vi "FTW-Test-Socket-Stress-InboxShutdown.vi"() -> (0 "Test Result":errorcluster)   [LabVIEW 2015]
panel:
  out "Endpoints":string[](array[string])
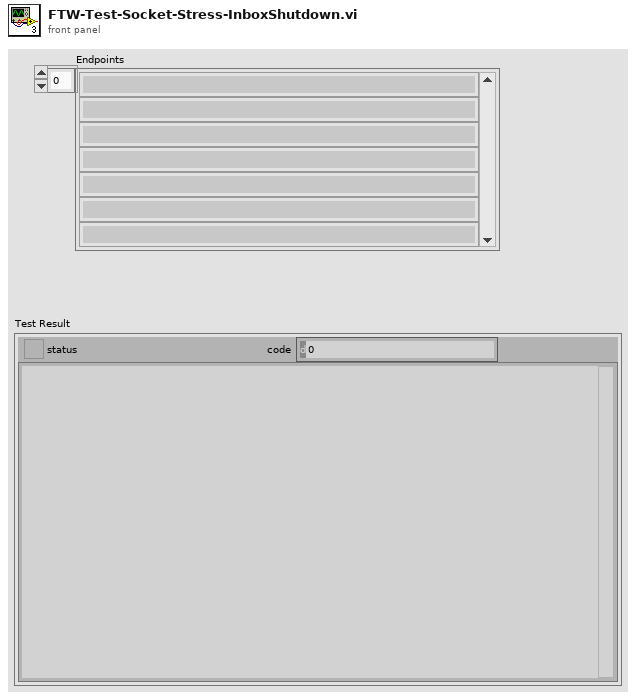
[diagram p1: front panel]
types:
  T1 = typedef "FTW-Type-Actor-Inbox.ctl" = refnum<data-value>
  T2 = cluster{"[0]":refnum<event-registration>, "[1]":refnum<event-registration>, "[2]":refnum<event-registration>, "[3]":refnum<event-registration>, "[4]":refnum<event-registration>, "[5]":refnum<event-registration>, "[6]":refnum<event-registration>, "[7]":refnum<event-registration>, "[8]":refnum<event-registration>, "[9]":refnum<event-registration>, "[10]":refnum<event-registration>, "[11]":refnum<event-registration>, "[12]":refnum<event-registration>, "[13]":refnum<event-registration>, "[14]":refnum<event-registration>, "[15]":refnum<event-registration>, "[16]":refnum<event-registration>, "[17]":refnum<event-registration>, "[18]":refnum<event-registration>, "[19]":refnum<event-registration>}
  T3 = typedef "FTW-Reflection-Types.ctl" = enum16{"Unknown", "Void", "Array", "Cluster", "LVObject", "Boolean", "I8", "I16", "I32", "I64", "U8", "U16", "U32", "U64", "SGL", "DBL", "EXT", "CSG", "CDB", "CXT", "FXP", "EnumU8", "EnumU16", "EnumU32", "EnumU64", "SGLwithUnit", "DBLwithUnit", "EXTwithUnit", "CSGwithUnit", "CDBwithUnit", "CXTwithUnit", "String", "Path", "Picture", "Tag", "LVVariant", "Timestamp", "WaveformI8", "WaveformI16", "WaveformI32", "WaveformI64", "WaveformU8", "WaveformU16", "WaveformU32", "WaveformU64", "WaveformSGL", "WaveformDBL", "WaveformEXT", "WaveformCSG", "WaveformCDB", "WaveformCXT", "WaveformDigital", "WaveformUnknownType", "DigitalData", "DynamicData", "ExternalData", "FileByteStream", "TDMStream", "dotNET", "ActiveX", "VIServerReference", "VIReference", "ApplicationInstance", "Menu", "ConnectionDataSocket", "ConnectionVISA", "ConnectionBluetooth", "ConnectionIrDA", "ConnectionTCP", "ConnectionUDP", "ConnectionHTTPClient", "ConnectionFTP", "Occurrence", "Notifier", "Queue", "Rendezvous", "Semaphore", "RTFIFO", "EventPublisher", "EventRegistration", "EventCallback", "DataValueReference", "GenericClass", "GenericClassTag", "GenericClassDeepCopy", "GenericClassFlattened", "GenericClassTagFlattened", "GenericReferenceType", "WindowsRegistry", "OverloadedDatalogRef", "ReferenceUnknownType", "ByteArray", "ConPaneInterface", "FTWObject"}
  T4 = cluster{"Element Name":string, "Element Type":T3, "Element Value":variant}[]
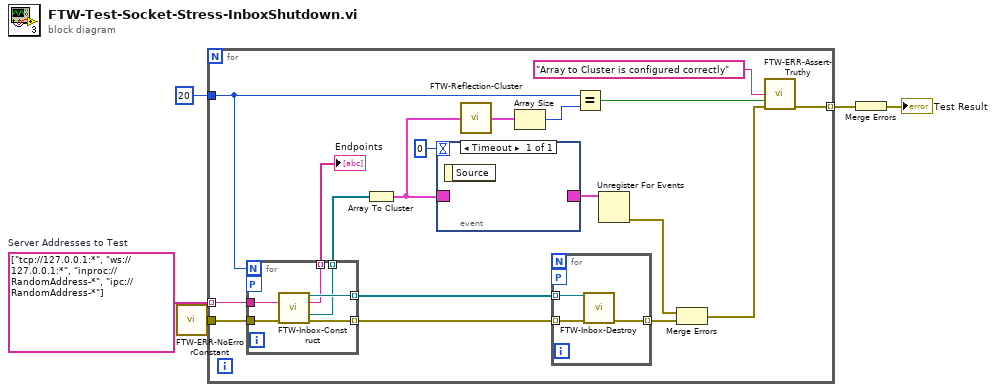
[diagram p0: block diagram]
diagram:
  w5 = string[] ["tcp://127.0.0.1:*", "ws://127.0.0.1:*", "inproc://RandomAddress-*", "ipc://RandomAddress-*"]  # Server Addresses to Test
  n1 = call "FTW-ERR-NoErrorConstant.vi"() -> ("no error"=w1:errorcluster)
  n2 = for {
    tunnel: [w9] -> w3 mode=indexing
    tunnel: w5 -> [w16] mode=indexing
    tunnel: 20 -> [w12]
    tunnel: w1 -> [w6]
    n3 = for {
      N: w12 -> [_]
      tunnel: [w32] -> w18 mode=indexing
      tunnel: [w31] -> w19 mode=indexing
      tunnel: [w27] -> w15 mode=indexing
      tunnel: [w30] -> w22 mode=indexing
      tunnel: w16 -> [w29]
      workers-P: _ -> [_]
      tunnel: w6 -> [w28]
      n4 = call "FTW-Inbox-Construct.vi"("Primary Inbox Address"=w29, "error in"=w28) -> ("FTW Actor Inbox"=w32:T1, "Resolved Primary Inbox Address"=w31:string, "Incoming Request"=w27:refnum<event-registration>, "error out"=w30:errorcluster)  [unwired: 8 in, 2 out]
    }
    "Endpoints" <- w19
    n5 = Array To Cluster(array=w15) -> (cluster=w7:T2)
    n6 = event shown="[0] Timeout" {
      selector: w7 -> [_]
      dyn-events: [_] -> w23
      timeout: 0 -> [_]
      event Timeout {
        n7 = event-data() -> ()  [unwired: 1 in, 1 out]
      }
    }
    n8 = call "FTW-Reflection-Cluster.vi"("Cluster"=w7) -> ("Cluster Elements"=w14:T4)  [unwired: 14 in]
    n9 = Array Size(array=w14) -> (size(s)=w13:i32)
    n10 = for {
      tunnel: w18 -> [w26] mode=indexing
      tunnel: w22 -> [w25] mode=indexing
      tunnel: [w24] -> w21 mode=indexing
      workers-P: _ -> [_]
      n11 = call "FTW-Inbox-Destroy.vi"("FTW Inbox"=w26, "error in"=w25) -> ("error out"=w24:errorcluster)  [unwired: 13 in]
    }
    n12 = Equal?(x=w12, y=w13) -> (x = y?=w8:bool)
    n13 = Unregister For Events(event registration refnum=w23) -> (error out=w17:errorcluster)  [unwired: 1 in]
    n14 = Merge Errors(w17, w21) -> (w10:errorcluster)
    n15 = call "FTW-ERR-Assert-Truthy.vi"("Assertion"="Array to Cluster is configured correctly", "Assertion holds true?"=w8, "error in"=w10) -> ("error out"=w9:errorcluster)  [unwired: 12 in]
  }
  n16 = Merge Errors(w3) -> (→"Test Result":errorcluster)
